vi "2转10进制字符串.vi"(1 "二进制字符串":string) -> (0 "十进制数值":i32)   [LabVIEW 2018]
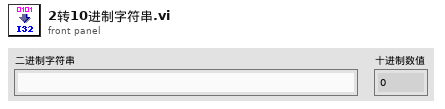
[diagram p1: front panel]
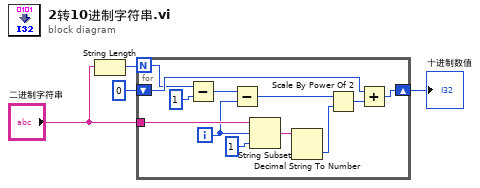
[diagram p0: block diagram]
diagram:
  n1 = String Length(string="二进制字符串") -> (length=w4:i32)
  n2 = for {
    N: w4 -> [w7]
    tunnel: "二进制字符串" -> [w14]
    shift-right: [w9] -> w1
    shift-left: 0 -> [w11]
    i -> [w13]
    n3 = Subtract(x=w7, y=1) -> (x-y=w8:i32)
    n4 = Subtract(x=w8, y=w13) -> (x-y=w12:i32)
    n5 = String Subset(string=w14, offset (0)=w13, length (rest)=1 ("长度（剩余）")) -> (substring=w15:string)
    n6 = Decimal String To Number(string=w15) -> (number=w5:i32)  [unwired: 2 in, 1 out]
    n7 = Scale By Power Of 2(n=w12, x=w5) -> (x*2^n=w10:i32)
    n8 = Add(x=w11, y=w10) -> (x+y=w9:i32)
  }
  "十进制数值" <- w1
